vi "Close Front Panel.vi"(0 "vi path":path, 5 "error in (no error)":errorcluster) -> (19 "error out":errorcluster)   [LabVIEW 2018]
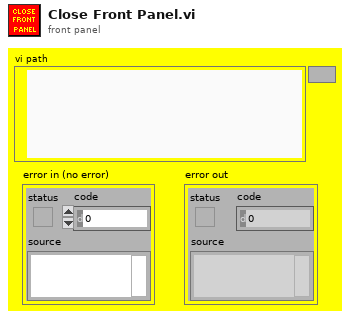
[diagram p1: front panel]
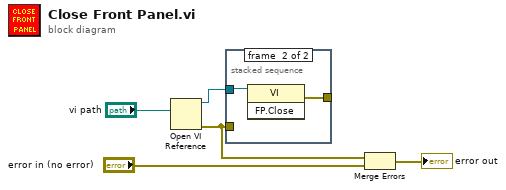
[diagram p0: block diagram]
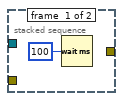
[diagram p2: hidden frame]
diagram:
  n1 = Open VI Reference(vi path="vi path") -> (vi reference=w4:refnum<vi>, error out=w2:errorcluster)  [unwired: 1 in, 4 out]
  n2 = stacked-sequence {
    tunnel: w2 -> [_ _]
    tunnel: w4 -> [_ w8]
    tunnel: [_ w7] -> _
    frame #0 {
      n3 = Wait (ms)(milliseconds to wait=u32 100) -> ()  [unwired: 1 out]
    }
    frame #1 {
      n4 = invoke class="VI" method="FP.Close"(reference=w8) -> (error out=w7:errorcluster)  [unwired: 2 in, 2 out]
    }
  }
  n5 = Merge Errors(w2, "error in (no error)") -> (→"error out":errorcluster)
